vi "Threshold ALERT.vi"(8 "error in (no error)":errorcluster, 11 "Alert Data":T1={"Tag"="", "Value"=0.0, "Alerts"=[FALSE, FALSE, FALSE], "Thresh Val"=0.0, "Thresh Len"=0.0, "Thresh Type"=enum."Neither"}) -> (0 "error out":errorcluster)   [LabVIEW 2018, in "RT - Analysis.lvlib"]
doc: "This subVI enqueues the named action in to the communications queue along with the input data."
uses:
  RT - Analysis.lvlib
  Public Controls/Alert Data.ctl
  Private Controls/Module Data.ctl
  Private Controls/Module Action.ctl
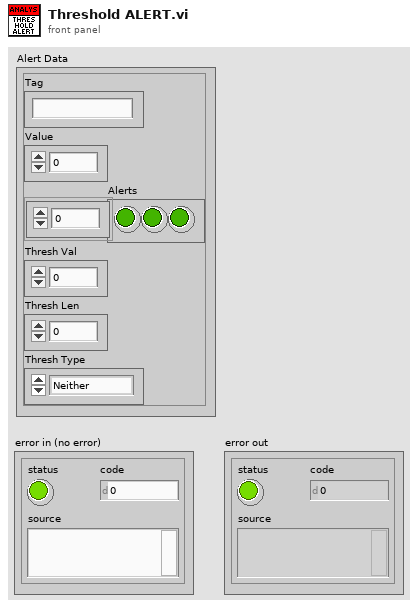
[diagram p1: front panel]
types:
  T1 = typedef "RT - Analysis.lvlib/Alert Data.ctl" = cluster{"Tag":string, "Value":dbl, "Alerts":bool[], "Thresh Val":dbl, "Thresh Len":dbl, "Thresh Type":enum16{"Neither", "Max", "Min"}}
  T2 = typedef "RT - Analysis.lvlib/Module Data.ctl" = cluster{"Data":variant, "Action":T3}
  T3 = typedef "RT - Analysis.lvlib/Module Action.ctl" = enum16{"Raw Data", "Set Repair Level", "APU Setup Info", "Init", "Error", "Set Highpass", "Threshold ALERT", "Set Accel Sens"}
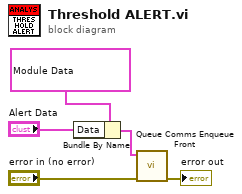
[diagram p0: block diagram]
diagram:
  n1 = Bundle By Name(cluster=T2 {"Data"=variant, "Action"=enum."Threshold ALERT"} ("element"), "Data"="Alert Data") -> (w4:T2)
  n2 = call "Queue Comms Enqueue Front.vi"("error in (no error)"="error in (no error)", "element"=w4) -> ("error out"=→"error out":errorcluster)  [unwired: 9 in]
